vi "Read Origin.vi"(8 "error in (no error)":errorcluster, 11 "Pane in":refnum<class "Pane.lvclass">) -> (0 "error out":errorcluster, 2 "Origin":T1, 3 "Pane out":refnum<class "Pane.lvclass">)   [LabVIEW 2017, in "Pane.lvclass"]
uses:
  Pane.lvclass
  Typedefs/Point--Cluster.ctl
  Pane.lvclass/Pane.ctl
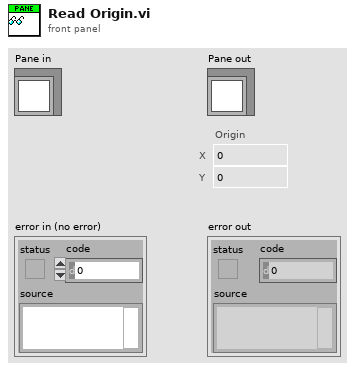
[diagram p1: front panel]
types:
  T1 = typedef "Point--Cluster.ctl" = cluster{"Horizontal":i32, "Vertical":i32}
  T2 = typedef "LVPointTypeDef.ctl" = cluster{"Horizontal":i16, "Vertical":i16}
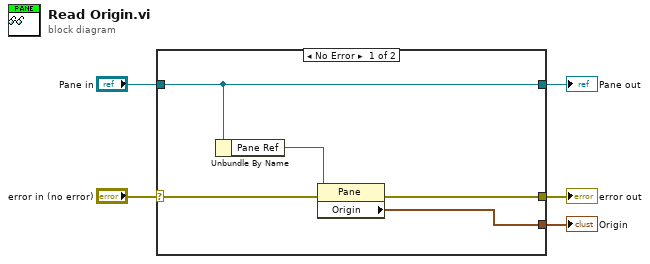
[diagram p0: block diagram]
diagram:
  n1 = case shown="No Error" "error in (no error)" {
    selector: "error in (no error)" -> [w10 w11]
    tunnel: [w8 w11] -> w4
    tunnel: [w9 w12] -> w2
    tunnel: "Pane in" -> [w9 w12]
    tunnel: [w6 _] -> w1
    frame No Error {
      n2 = Unbundle By Name(w9) -> ("Pane Ref"=w7:refnum<vi>)
      n3 = property class="Pane"(reference=w7, error in=w10) -> (error out=w8:errorcluster, "Origin"=w6:T2)  [unwired: 1 out]
    }
    frame Error {
    }
  }
  "error out" <- w4
  "Pane out" <- w2
  "Origin" <- w1
